vi "Control ITC Sweep -- running averages.vi"(5 "seconds":i32=6, 7 "history length (sec)":i32=7200, 9 "more state":T1={"time(min)"=0.0, "T (ITC )"=300.0, "T (ITC, set)"=295.0, "heater"=0.0, "gas"=99.9, "T (ITC)  - T (ITC, set)"=5.420000000368873, "T (LTC)  - T (ITC, set)"=5.718000000368875, "heater slope"=-38.40000000008513, "LTC slope"=55.45200000012313, "hetaer running average"=-1.9200000000055297, "T (LTC)"=300.298, "T (LTC) running average"=303.0705999999136}, 10 "thermometer reading":T3={"LTC21 Address"="GPIB0::15::INSTR", "ITC503 Address"="GPIB0::24::INSTR", "ITC temperature"=300.0, "ITC set temperature"=295.0, "LTC temperature"=300.297, "heater"=0.0, "gas flow"=99.9, "P"=10.0, "D"=1.0, "I"=3.0, "ITC state"="X0A1C2S01H1L0\r", "nonzero temperature"=0.0}, 11 "more state -- aggregate":T2={"time(min)"=array[7200 elements], "T (ITC )"=array[7200 elements], "T (ITC, set)"=array[7200 elements], "T (LTC)"=array[7200 elements], "heater"=array[7200 elements], "gas"=array[7200 elements], "T (ITC)  - T (ITC, set)"=array[7200 elements], "T (LTC)  - T (ITC, set)"=array[7200 elements], "heater slope"=array[7200 elements], "LTC slope"=array[7200 elements], "hetaer running average"=array[7200 elements], "T (LTC) running average"=array[7200 elements]}) -> (2 "more state out":T1={"time(min)"=0.0, "T (ITC )"=300.0, "T (ITC, set)"=295.0, "heater"=0.0, "gas"=99.9, "T (ITC)  - T (ITC, set)"=5.420000000368873, "T (LTC)  - T (ITC, set)"=5.718000000368875, "heater slope"=-38.40000000008513, "LTC slope"=55.45200000012313, "hetaer running average"=-1.9200000000055297, "T (LTC)"=300.298, "T (LTC) running average"=303.0705999999136})   [LabVIEW 2010]
uses:
  state.ctl
  collect.ctl
  collect - input.ctl
  <vilib>/Analysis/6fits.llb/Curve Fitting Criteria.ctl
  <vilib>/Analysis/NI_AALPro.lvlib
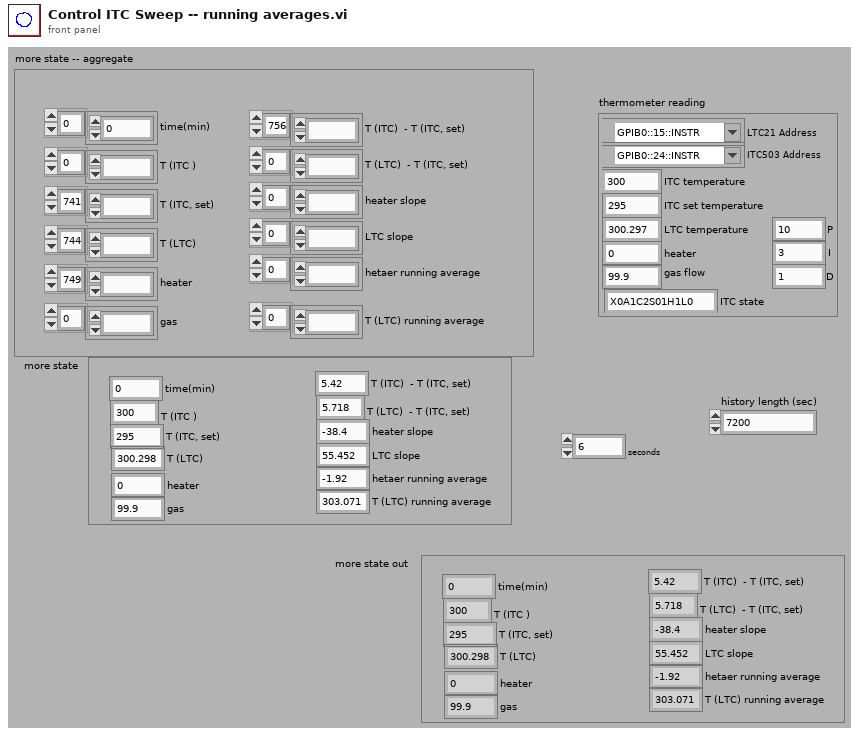
[diagram p1: front panel]
types:
  T1 = typedef "collect - input.ctl" = cluster{"time(min)":dbl, "T (ITC )":dbl, "T (ITC, set)":dbl, "heater":dbl, "gas":dbl, "T (ITC)  - T (ITC, set)":dbl, "T (LTC)  - T (ITC, set)":dbl, "heater slope":dbl, "LTC slope":dbl, "hetaer running average":dbl, "T (LTC)":dbl, "T (LTC) running average":dbl}
  T2 = typedef "collect.ctl" = cluster{"time(min)":dbl[], "T (ITC )":dbl[], "T (ITC, set)":dbl[], "T (LTC)":dbl[], "heater":dbl[], "gas":dbl[], "T (ITC)  - T (ITC, set)":dbl[], "T (LTC)  - T (ITC, set)":dbl[], "heater slope":dbl[], "LTC slope":dbl[], "hetaer running average":dbl[], "T (LTC) running average":dbl[]}
  T3 = typedef "state.ctl" = cluster{"LTC21 Address":refnum<visa-resource-name>, "ITC503 Address":refnum<visa-resource-name>, "ITC temperature":dbl, "ITC set temperature":dbl, "LTC temperature":dbl, "heater":dbl, "gas flow":dbl, "P":dbl, "D":dbl, "I":dbl, "ITC state":string, "nonzero temperature":dbl}
  T4 = typedef "NI_AALPro.lvlib/Curve Fitting Criteria.ctl" = u16
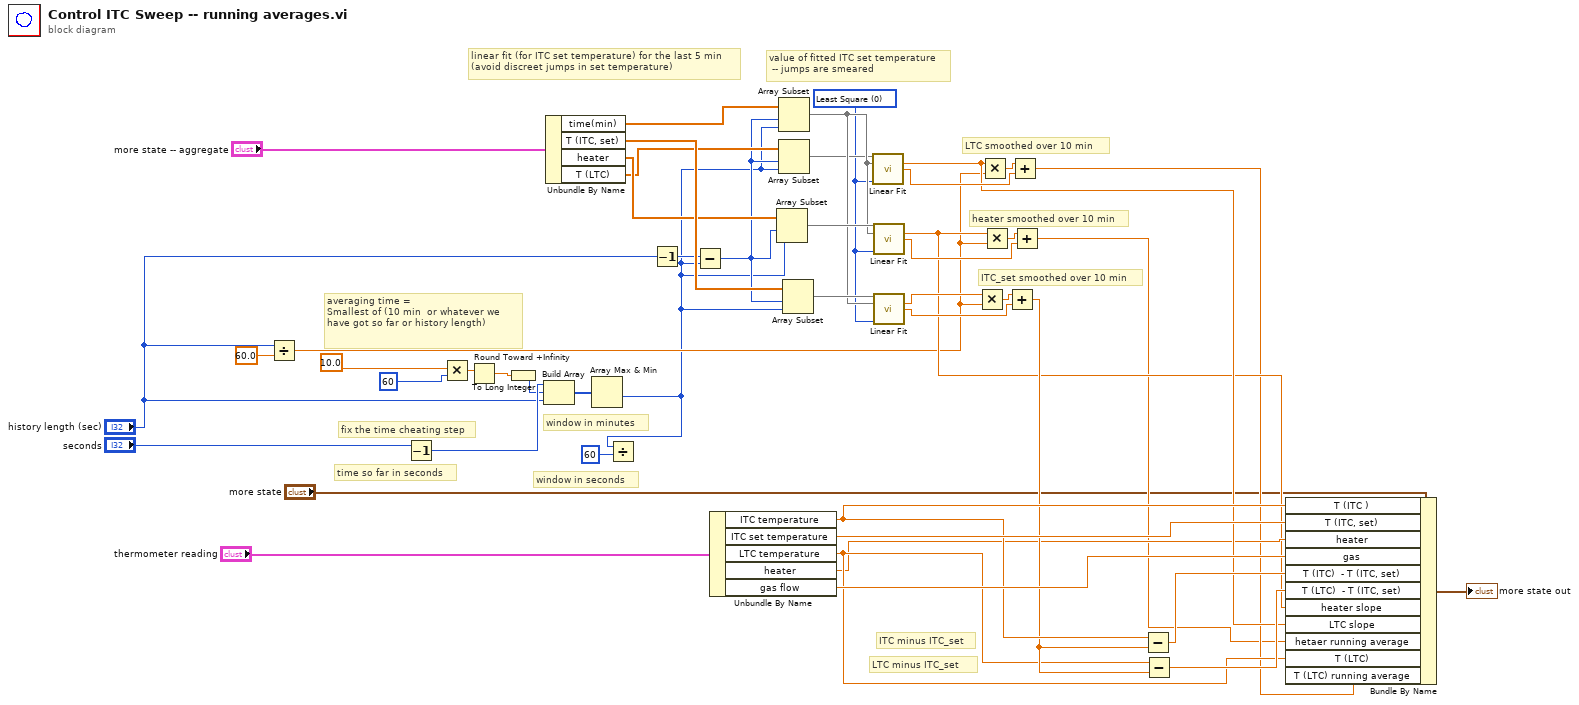
[diagram p0: block diagram]
diagram:
  w22 = T4 0 items=["Least Square", "Least Absolute Residual", "Bisquare"] ("method")
  # "LTC minus ITC_set"
  # "ITC minus ITC_set"
  # "ITC_set smoothed over 10 min"
  # "LTC smoothed over 10 min"
  # "heater smoothed over 10 min"
  # "window in minutes"
  # "window in seconds"
  # "time so far in seconds"
  # "fix the time cheating step"
  # "value of fitted ITC set temperature\n -- jumps are smeared"
  # "averaging time =\nSmallest of (10 min  or whatever we have got so far or history length)"
  # "linear fit (for ITC set temperature) for the last 5 min\n(avoid discreet jumps in set temperature)"
  n1 = Divide(x="history length (sec)", y=60.0) -> (x/y=w5:dbl)
  n2 = Decrement(x="seconds") -> (x-1=w30:i32)
  n3 = Multiply(x=10.0 ("standard deviation"), y=60) -> (x*y=w47:dbl)
  n4 = Round Toward +Infinity(x=w47) -> (ceil(x): smallest int >= x=w46:dbl)
  n5 = To Long Integer(number=w46) -> (32bit integer=w29:i32)
  n6 = Build Array(w30, w29, "history length (sec)") -> (w28:i32[])
  n7 = Unbundle By Name("more state -- aggregate") -> ("time(min)"=w26:dbl[], "T (ITC, set)"=w35:dbl[], "heater"=w33:dbl[], "T (LTC)"=w32:dbl[])
  n8 = Array Max & Min(array=w28) -> (min value=w1:i32)  [unwired: 3 out]
  n9 = Divide(x=w1, y=60) -> ()  [unwired: 1 out]
  n10 = Decrement(x="history length (sec)") -> (x-1=w27:i32)
  n11 = Subtract(x=w27, y=w1) -> (x-y=w25:i32)
  n12 = Unbundle By Name("thermometer reading") -> ("ITC temperature"=w19:dbl, "ITC set temperature"=w21:dbl, "LTC temperature"=w15:dbl, "heater"=w13:dbl, "gas flow"=w20:dbl)
  n13 = Array Subset(array=w33, index=w25, length=w1) -> (w31:dbl[])
  n14 = Array Subset(array=w26, index=w25, length=w1) -> (w24:dbl[])
  n15 = Array Subset(array=w32, index=w25, length=w1) -> (w23:dbl[])
  n16 = Array Subset(array=w35, index=w25, length=w1) -> (w34:dbl[])
  n17 = call <vilib>:"Linear Fit.vi"("Y"=w23, "X"=w24, "method"=w22) -> ("slope"=w14:dbl, "intercept"=w36:dbl)  [unwired: 8 in, 3 out]
  n18 = call <vilib>:"Linear Fit.vi"("Y"=w31, "X"=w24, "method"=w22) -> ("slope"=w12:dbl, "intercept"=w38:dbl)  [unwired: 8 in, 3 out]
  n19 = call <vilib>:"Linear Fit.vi"("Y"=w34, "X"=w24, "method"=w22) -> ("slope"=w42:dbl, "intercept"=w41:dbl)  [unwired: 8 in, 3 out]
  n20 = Multiply(x=w42, y=w5) -> (x*y=w43:dbl)
  n21 = Multiply(x=w14, y=w5) -> (x*y=w37:dbl)
  n22 = Multiply(x=w12, y=w5) -> (x*y=w39:dbl)
  n23 = Add(x=w43, y=w41) -> (x+y=w18:dbl)
  n24 = Add(x=w37, y=w36) -> (x+y=w11:dbl)
  n25 = Add(x=w39, y=w38) -> (x+y=w10:dbl)
  n26 = Subtract(x=w19, y=w18) -> (x-y=w17:dbl)
  n27 = Subtract(x=w15, y=w18) -> (x-y=w16:dbl)
  n28 = Bundle By Name(cluster="more state", "T (ITC )"=w19, "T (ITC, set)"=w21, "heater"=w13, "gas"=w20, "T (ITC)  - T (ITC, set)"=w17, "T (LTC)  - T (ITC, set)"=w16, "heater slope"=w12, "LTC slope"=w14, "hetaer running average"=w10, "T (LTC)"=w15, "T (LTC) running average"=w11) -> (→"more state out":T1)
